vi "RT-Motor-Controls.vi"(0 "Settings":T4) -> (3 "Error":T3)   [LabVIEW 2020]
uses:
  <vilib>/RioEmbeddedCAN/RioEmbeddedCAN.llb/CANFrameControl.ctl
panel:
  in  "U64-Input":u64(slide) scale=0.0..1.8446744073709552e+19
  out "CAN output":T1 {"type" items=["CAN Data", "CAN Remote"]; "identifier" format="%.0x"}
  out "Frames":string[][](table)
  out "CAN input":T2
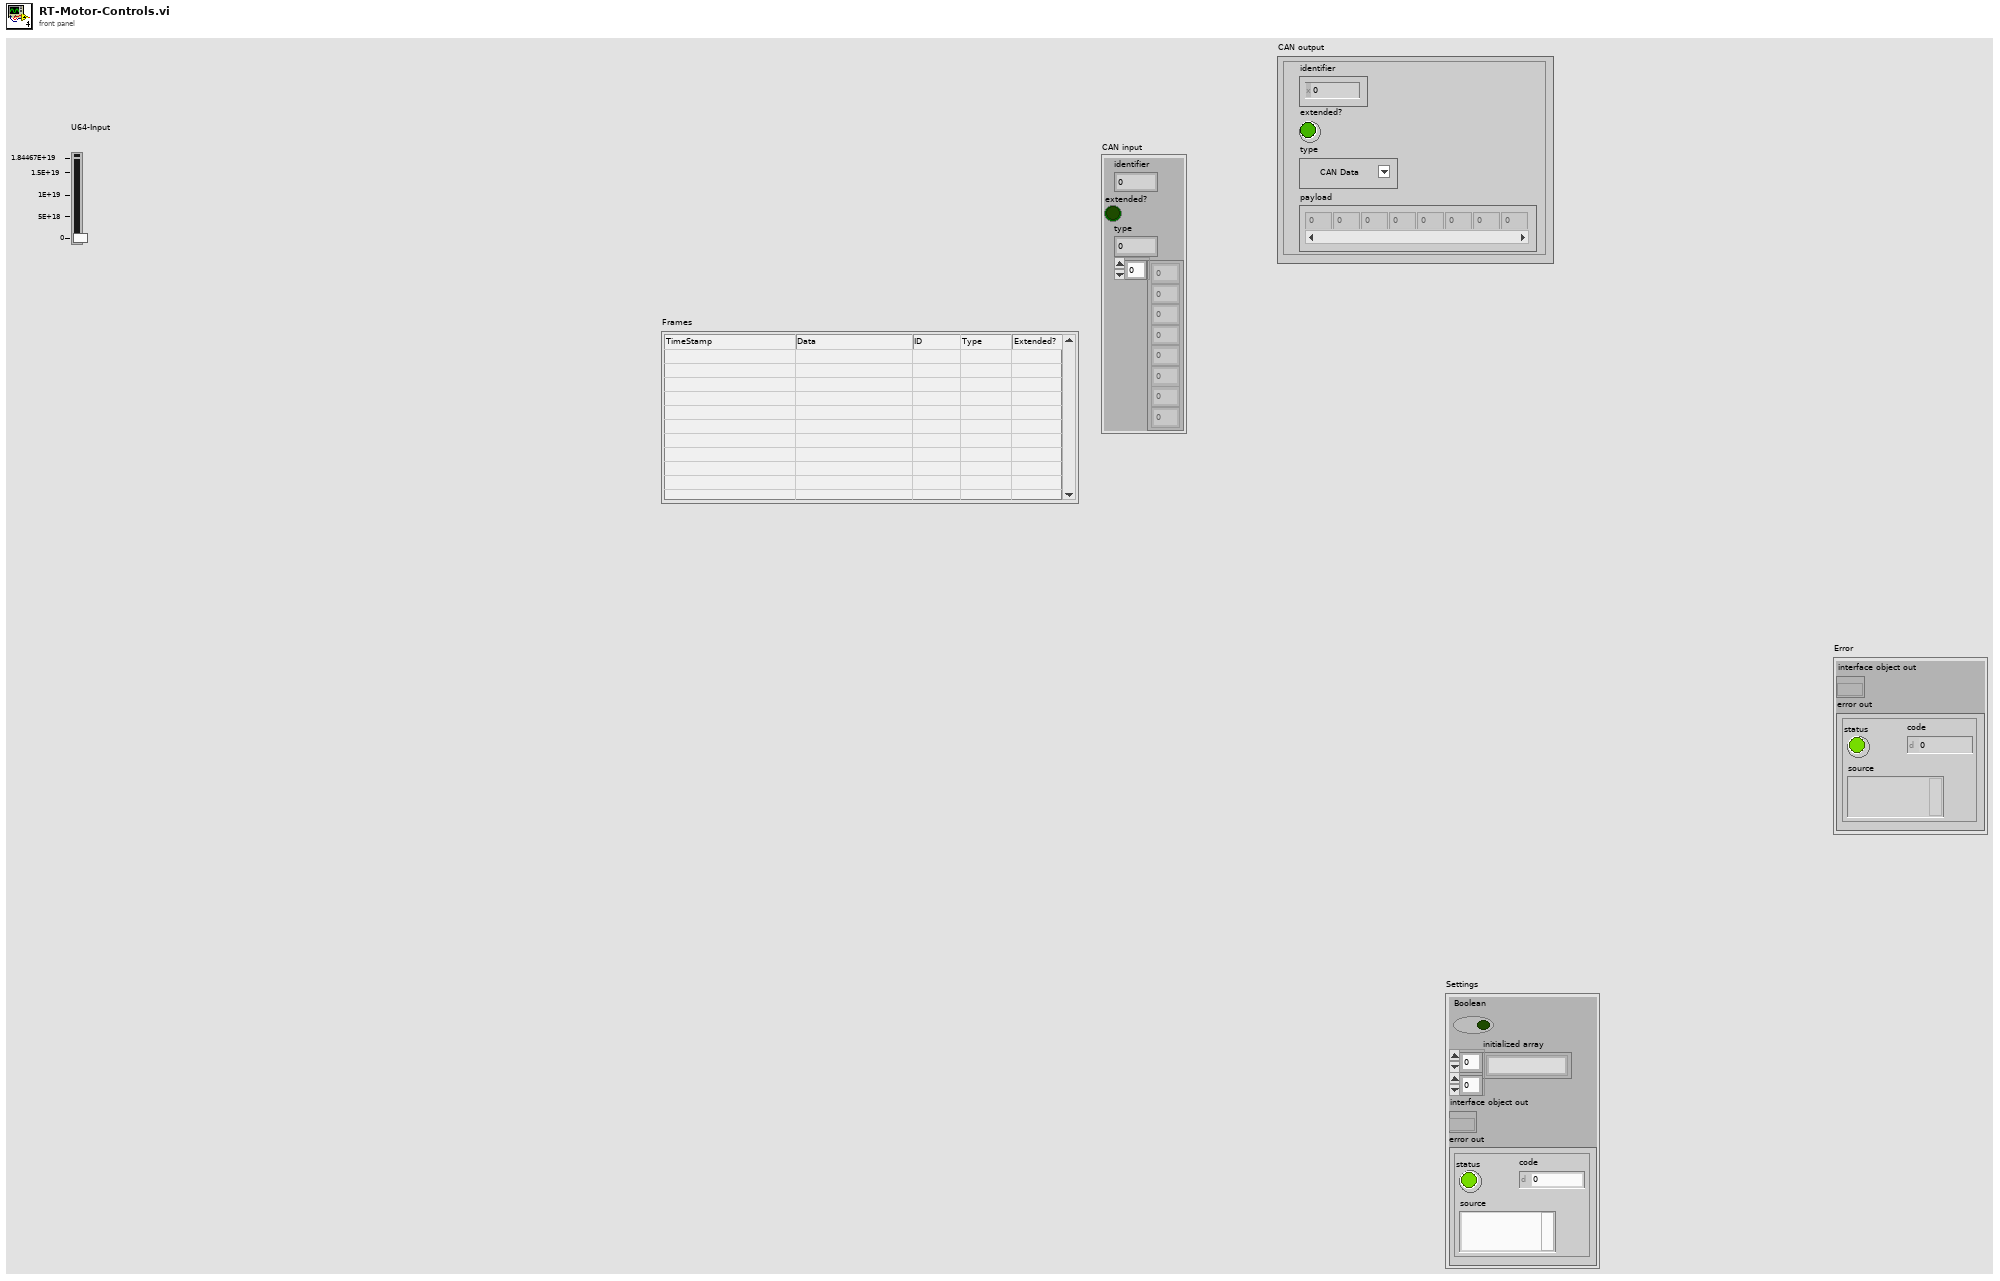
[diagram p1: front panel]
types:
  T1 = typedef "CANFrameControl.ctl" = cluster{"identifier":u32, "extended?":bool, "type":u8, "payload":u8[]}
  T2 = cluster{"identifier":u32, "extended?":bool, "type":u8, u64[]}
  T3 = cluster{"interface object out":refnum<k20>, "error out":errorcluster}
  T4 = cluster{"Boolean":bool, "initialized array":string[][], "interface object out":refnum<k20>, "error out":errorcluster}
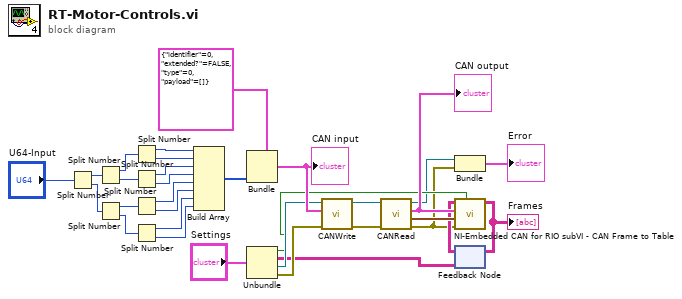
[diagram p0: block diagram]
diagram:
  n1 = Split Number(x="U64-Input") -> (hi(x)=w27:u32, lo(x)=w26:u32)
  n2 = Split Number(x=w27) -> (hi(x)=w25:u16, lo(x)=w24:u16)
  n3 = Split Number(x=w26) -> (hi(x)=w23:u16, lo(x)=w22:u16)
  n4 = Split Number(x=w25) -> (hi(x)=w14:u8, lo(x)=w15:u8)
  n5 = Split Number(x=w24) -> (hi(x)=w16:u8, lo(x)=w17:u8)
  n6 = Split Number(x=w23) -> (hi(x)=w18:u8, lo(x)=w19:u8)
  n7 = Split Number(x=w22) -> (hi(x)=w20:u8, lo(x)=w21:u8)
  n8 = Build Array(w14, w15, w16, w17, w18, w19, w20, w21) -> (w13:u8[])
  n9 = Bundle(cluster=T1 {"identifier"=0, "extended?"=FALSE, "type"=0, "payload"=[]} ("CAN frame"), "payload"=w13) -> (w11:T1)  [unwired: 3 in]
  "CAN input" <- w11
  n10 = Unbundle("Settings") -> ("Boolean"=w3:bool, "initialized array"=w4:string[][], "interface object out"=w7:refnum<k20>, "error out"=w8:errorcluster)
  n11 = call <vilib>:"CANWrite.vi"("error in (no error)"=w8, "CAN frame"=w11, "interface object in"=w7) -> ("error out"=w9:errorcluster, "interface object out"=w10:refnum<k20>)  [unwired: 7 in]
  n12 = call <vilib>:"CANRead.vi"("error in (no error)"=w9, "interface object in"=w10) -> ("error out"=w1:errorcluster, "timestamp"=w30:timestamp, "CAN frame"=w29:T1, "interface object out"=w2:refnum<k20>)  [unwired: 6 in]
  "CAN output" <- w29
  n13 = Bundle("interface object out"=w2, "error out"=w1) -> (→"Error":T3)  [unwired: 1 in]
  n14 = feedback #1(w4) -> (w6:string[][])
  n15 = call "NI-Embedded CAN for RIO subVI - CAN Frame to Table.vi"("Hexadecimal?"=w3, "error in (no error)"=w1, "timestamp"=w30, "CAN frame"=w29, "Input Array"=w6) -> ("Output Array"=w5:string[][])  [unwired: 6 in]
  "Frames" <- w5
  n16 = feedback-in #1(w5) -> ()
